vi "Read Parameter.vi"(8 "error in (no error)":errorcluster, 11 "ADOMapper in":refnum<class "ADOMapper.lvclass">) -> (0 "error out":errorcluster, 2 "DynamicParameters out":refnum<class "DynamicParameters.lvclass">, 3 "ADOMapper out":refnum<class "ADOMapper.lvclass">)   [LabVIEW 2020, in "ORM_ADONet.lvlib" / "ADOMapper.lvclass"]
uses:
  ADOMapper.lvclass
  <vilib>/Viviota/shared/ORM.lvlibp/ORM/DynamicParameters/DynamicParameters.lvclass
  ADOParameter/ADOParameter.lvclass
  C:/Program Files/National Instruments/LabVIEW 2020/vi.lib/Viviota/shared/ORM.lvlibp/ORM/DynamicParameters/DynamicParameters.lvclass
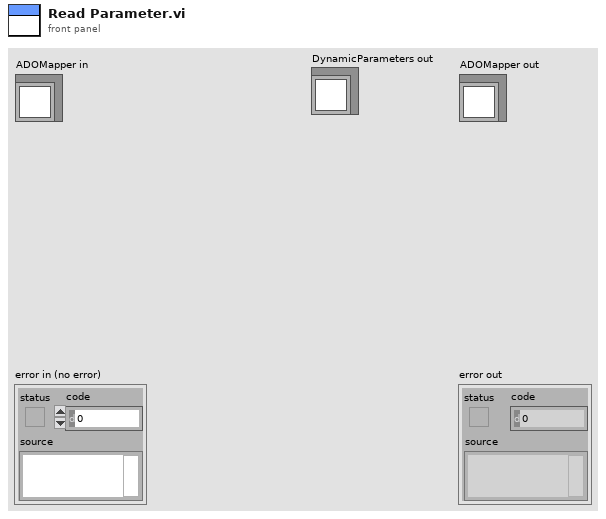
[diagram p1: front panel]
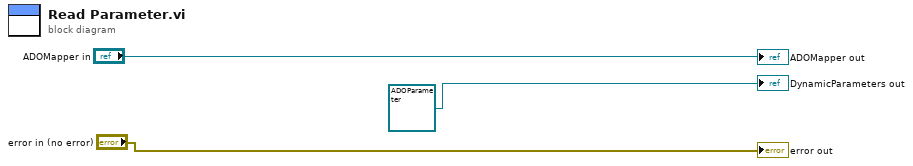
[diagram p0: block diagram]
diagram:
  "error out" <- "error in (no error)"
  "ADOMapper out" <- "ADOMapper in"
  "DynamicParameters out" <- refnum<class "ADOParameter.lvclass"> refnum ("ADONet.lvlib:ADOParameter.lvclass")
